vi "TEST X Graph Simple XControl.vi"() -> ()   [LabVIEW 2011]
doc: "This tests a simple X control that could be used in an introductory session on X Controls. \n\nAAL 9/09"
uses:
  Xgraph simple.xctl
panel:
  in  "show points":bool
  in  "stop":bool
  out "Xgraph simple":dbl[][](xcontrol)=[[0.8605863431398226, 0.19758562175436634, 0.7170782592970553, 0.39438832172355287, 0.794343689326255, 0.9455700387052649, 0.04446541111238078, 0.7361994452261094, 0.09184967366868424, 0.06532681565659582, 0.9496912231081271, 0.6350047940565837, 0.6353414643599069, 0.142816544846061, 0.21142560680398104, 0.04384741284704452, 0.2535348307632717, 0.17166259113565063, 0.2986167732922004, 0.8997946863698456, 0.15626926746563585, 0.1877884077433707, 0.5064092345214781, 0.20133212372898956, 0.6027619430748128, 0.3892958141781433, 0.897512160405423, 0.44217873924659923, 0.9186814327486243, 0.18272434060153953, 0.5483257192145732, 0.25748814052326296, 0.8746564693808243, 0.853207444482253, 0.08275392987299268, 0.7224840491310457, 0.6447899301516902, 0.9909984510219392, 0.26496980130532144, 0.0057431797563034515, 0.16038884561621103, 0.0815818774339796, 0.34969668530752296, 0.5125821782531186, 0.5124738929405841, 0.5796713851438011, 0.5311367679140169, 0.5035729921181928, 0.06596441415930876, 0.49477067245404704], [0.7810534687254789, 1.553317648545896, 1.5857644340213535, 1.9521550531470793, 1.4032964642467354, 0.5461981182045403, 1.5791355082939629, 0.9582828616921177, 1.112996914009881, 1.18511367736114, 0.2878007660679329, 0.18971348366818708, 0.6555689042333297, 1.6030038372890125, 1.5324316544979575, 0.17874690775963264, 1.034166364030435, 0.060858223356706986, 1.7671575774318207, 1.1335746622108829, 0.47790670720184947, 0.3030845305266259, 1.2042359008140258, 1.2441077957664106, 1.0216223690266433, 0.14172125128666213, 0.6886900387948103, 1.9364125109298622, 0.037318311491195466, 0.9075856082408715, 1.965646143876181, 0.2019341394277454, 1.5258091075032871, 0.018719928654225004, 1.3512992993400186, 1.636839890896686, 1.4137955962083368, 0.9569036817689676, 0.8423772242128695, 1.1676094150538643, 0.6537596289976566, 0.1617356352651682, 1.6478518811575031, 1.8699917445941119, 1.088797328482518, 0.45707298859581513, 0.5218343491383766, 0.5386212356884545, 1.1858174109419726, 0.011360598055938809], [1.9145337761615353, 1.0253626246376166, 2.4461694208515277, 0.4869131571667298, 0.050206757099168, 1.7111278845485636, 2.833818455592326, 1.9823454711275348, 2.5885234155274164, 0.2337937671435959, 1.1346021671623026, 2.8126440848300023, 2.5025763703780086, 0.2771667464061389, 0.11209201108544176, 1.8368183040565094, 2.1710940927519555, 2.93510878970066, 2.9878194377872824, 1.4456449502315842, 1.4719927787917977, 2.967685228409313, 2.848936925703078, 2.9947065046136734, 2.6888960413171183, 2.345663893068195, 1.298369275356395, 1.4978377735868729, 0.1331017342636367, 0.26756807542237704, 0.09353492415957998, 0.3720914467644305, 2.8921299635392956, 0.41897309223222257, 0.6260147396923756, 0.4908596855709908, 2.7661082039305174, 0.5592224242508319, 2.399480823369192, 1.4881429990020842, 2.65072202148682, 2.036317457741897, 1.514417336069842, 0.1923803248160394, 2.714959707022886, 0.04451884410945528, 2.462040752486228, 0.8783657659220967, 0.46404935905433264, 1.2996642162677934], [3.138812136147334, 1.1611146195366633, 2.1974695291520474, 2.2384355756328773, 1.4376821232129622, 1.0299049424020144, 3.405610375853165, 1.8801151608819335, 3.453894708390096, 0.4895233739775122, 3.5828975536605436, 3.754771786425608, 3.7095467420610504, 1.9910347134587418, 1.6645004201135167, 2.4337564245156758, 0.41987482468818715, 2.0952980890726547, 2.1013837567116473, 1.1893314841148843, 2.7984319269374813, 3.8980374978472074, 0.6415753688037897, 1.0547425276377034, 0.2191504208366677, 2.8071901523419327, 2.6032211378900505, 3.9881001684070903, 1.1800441592162798, 3.057976438047679, 1.2742201338452226, 1.863678008901282, 3.4375333110965647, 1.5303232187035425, 2.3503219477924633, 2.7585833707831773, 1.5178114226895678, 1.9386482262042486, 0.2701695870743962, 2.3232038252032696, 2.663995279903257, 1.2857795729566401, 0.6651466105673141, 1.0238397988305579, 2.5348107288980923, 2.741771901188656, 3.8099696509115875, 3.8366344608330163, 3.2125804686542048, 3.458951200100537]]
  # "Show Points"
  # "Hide Points"
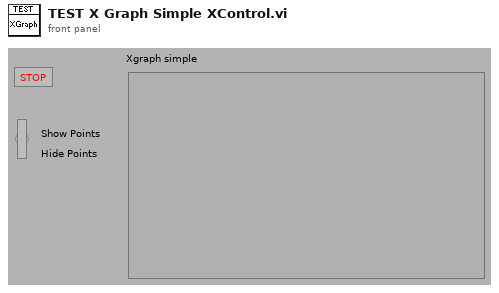
[diagram p1: front panel]
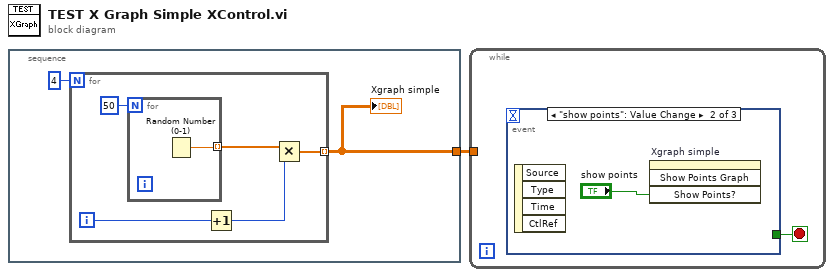
[diagram p0: block diagram]
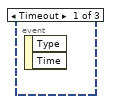
[diagram p2: hidden frame]
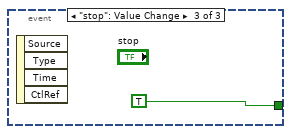
[diagram p3: hidden frame]
diagram:
  n1 = stacked-sequence {
    tunnel: [w2] -> w1
    frame #0 {
      n2 = for {
        N: 4 -> [_]
        tunnel: [w4] -> w2 mode=indexing
        i -> [w6]
        n3 = for {
          N: 50 -> [_]
          tunnel: [w9] -> w7 mode=indexing
          n4 = Random Number (0-1)() -> (number: 0 to 1=w9:dbl)
        }
        n5 = Increment(x=w6) -> (x+1=w5:i32)
        n6 = Multiply(x=w7, y=w5) -> (x*y=w4:dbl[])
      }
      "Xgraph simple" <- w2
    }
  }
  n7 = while {
    tunnel: w1 -> [_]
    stop <- w10 stop-if-true
    n8 = event shown="[1] \"show points\": Value Change" {
      selector: _ -> [_ _ _]
      dyn-events: _ -> [_ _ _]
      timeout: _ -> [_ _ _]
      tunnel: [_ _ TRUE] -> w10
      event Timeout {
        n9 = event-data() -> ()  [unwired: 1 in, 2 out]
      }
      event "show points": Value Change {
        n10 = event-data() -> ()  [unwired: 1 in, 4 out]
        n11 = invoke on="Xgraph simple" class="Xgraph simple (strict)" method="Show Points Graph"("Show Points?"="show points") -> ()  [unwired: 3 in, 4 out]
      }
      event "stop": Value Change {
        n12 = event-data() -> ()  [unwired: 1 in, 4 out]
      }
    }
  }
